vi "Configure Waveform (User Defined).vi"(0 "VISA resource name":refnum<visa-resource-name>, 1 "List Of Output Data Mode (1: New List)":i32(ring)=1 items=["Append", "New List"], 2 "Enable Trigger Output (T: Enable)":bool=TRUE, 3 "List Of Trigger Output Mode (1: New List)":i32(ring)=1 items=["Append", "New List"], 5 "Output Channel (0: Channel 1)":i32(ring) items=["Channel 1", "Channel 2"], 7 "Source Mode (1: Voltage)":i32(ring)=1 items=["Current", "Voltage"], 9 "Step Time (1E-5 seconds)":dbl=1e-05, 11 "error in (no error)":errorcluster, 12 "List Of Output Data":dbl[](array[numeric])=[0.0], 13 "Trigger Output Port (0: External1)":i32(ring) items=["External1", "External2", "External3", "External4", "External5", "External6", "External7", "External8", "External9", "External10", "External11", "External12", "External13", "External14", "Internal1", "Internal2"], 14 "List Of Trigger Output":bool[](array[boolean])=[FALSE]) -> (4 "VISA resource name out":refnum<visa-resource-name>, 15 "error out":errorcluster)   [LabVIEW 2023, in "Agilent B2900 Series.lvlib"]
doc: "Configure current or voltage user defined waveform output.\n\n<B>Note:</B>\nThis VI is only supported by Agilent models B2961A, B2962A, B2961B,B2962B,B2961C and B2962C."
uses:
  Agilent B2900 Series.lvlib
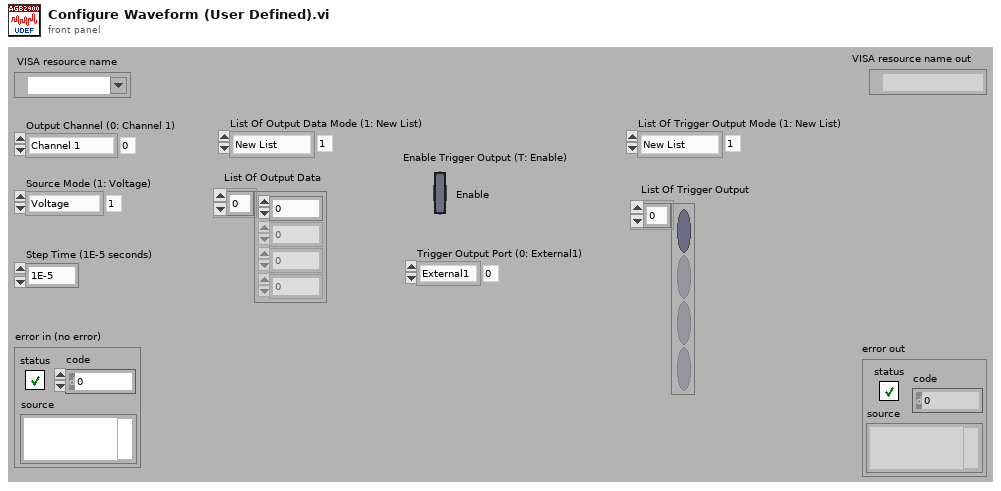
[diagram p1: front panel]
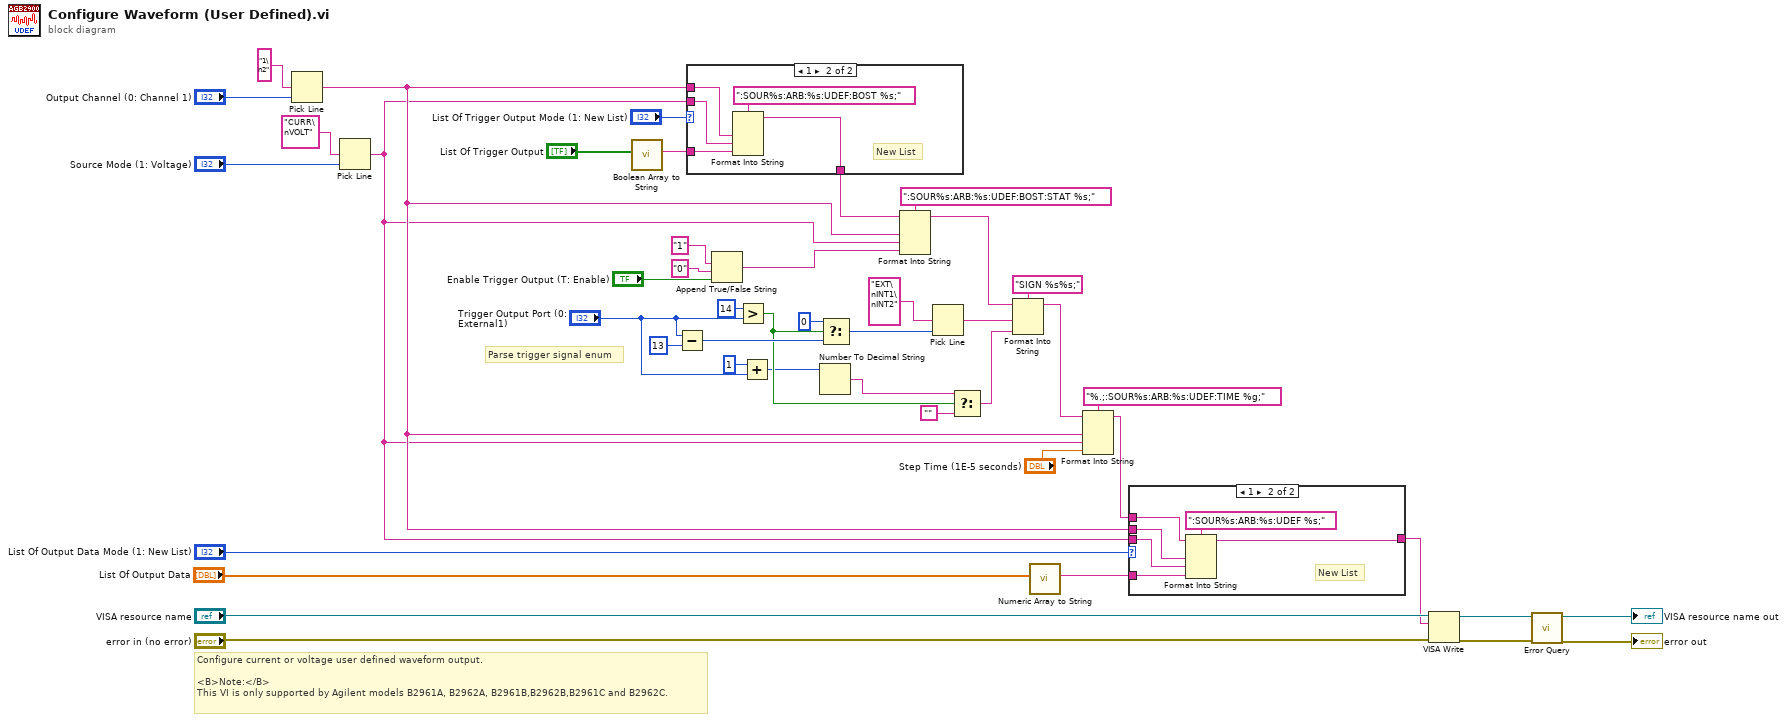
[diagram p0: block diagram]
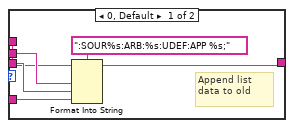
[diagram p2: hidden frame]
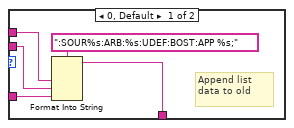
[diagram p3: hidden frame]
diagram:
  # "Parse trigger signal enum"
  # "Configure current or voltage user defined waveform output.\n\n<B>Note:</B>\nThis VI is only supported by Agilent models B2961A, B2962A, B2961B,B2962B,B2961C and B2962C."
  n1 = Pick Line(multi-line string="1\n2", line index="Output Channel (0: Channel 1)") -> (output string=w7:string)  [unwired: 1 in]
  n2 = Pick Line(multi-line string="CURR\nVOLT", line index="Source Mode (1: Voltage)") -> (output string=w6:string)  [unwired: 1 in]
  n3 = call "Boolean Array to String.vi"("List Data"="List Of Trigger Output") -> ("Result String"=w29:string)  [unwired: 10 in]
  n4 = Subtract(x="Trigger Output Port (0: External1)", y=13) -> (x-y=w23:i32)
  n5 = case shown="1" "List Of Trigger Output Mode (1: New List)" {
    tunnel: w7 -> [w49 w54]
    tunnel: w6 -> [w48 w53]
    tunnel: w29 -> [w47 w52]
    tunnel: [w46 w51] -> w9
    frame 0, Default {
      # "Append list data to old"
      n6 = Format Into String(format string=":SOUR%s:ARB:%s:UDEF:BOST:APP %s;", w49, w48, w47) -> (resulting string=w46:string)  [unwired: 2 in, 1 out]
    }
    frame 1 {
      # "New List"
      n7 = Format Into String(format string=":SOUR%s:ARB:%s:UDEF:BOST %s;", w54, w53, w52) -> (resulting string=w51:string)  [unwired: 2 in, 1 out]
    }
  }
  n8 = Append True/False String(1:"Enable Trigger Output (T: Enable)", 2:"0", 3:"1") -> (0:w10:string)  [unwired: 1 out]
  n9 = Greater?(x=14 ("y"), y="Trigger Output Port (0: External1)") -> (0:w20:bool)
  n10 = Add(x=1, y="Trigger Output Port (0: External1)") -> (x+y=w18:i32)
  n11 = Number To Decimal String(number=w18) -> (decimal integer string=w26:string)  [unwired: 1 in]
  n12 = Select(t=0, s=w20, f=w23) -> (s? t:f=w25:i32)
  n13 = Format Into String(format string=":SOUR%s:ARB:%s:UDEF:BOST:STAT %s;", initial string=w9, w7, w6, w10) -> (resulting string=w12:string)  [unwired: 1 in, 1 out]
  n14 = Pick Line(multi-line string="EXT\nINT1\nINT2", line index=w25) -> (output string=w14:string)  [unwired: 1 in]
  n15 = Select(t=w26, s=w20, f="") -> (s? t:f=w13:string)
  n16 = Format Into String(format string="SIGN %s%s;", initial string=w12, w14, w13) -> (resulting string=w11:string)  [unwired: 1 in, 1 out]
  n17 = call "Numeric Array to String.vi"("List Data"="List Of Output Data") -> ("Result String"=w16:string)  [unwired: 10 in]
  n18 = Format Into String(format string="%.;:SOUR%s:ARB:%s:UDEF:TIME %g;", initial string=w11, w7, w6, "Step Time (1E-5 seconds)") -> (resulting string=w8:string)  [unwired: 1 in, 1 out]
  n19 = case shown="1" "List Of Output Data Mode (1: New List)" {
    tunnel: w16 -> [w60 w64]
    tunnel: w7 -> [w59 w66]
    tunnel: w6 -> [w58 w65]
    tunnel: w8 -> [w57 w63]
    tunnel: [w56 w62] -> w1
    frame 0, Default {
      # "Append list data to old"
      n20 = Format Into String(format string=":SOUR%s:ARB:%s:UDEF:APP %s;", initial string=w57, w59, w58, w60) -> (resulting string=w56:string)  [unwired: 1 in, 1 out]
    }
    frame 1 {
      # "New List"
      n21 = Format Into String(format string=":SOUR%s:ARB:%s:UDEF %s;", initial string=w63, w66, w65, w64) -> (resulting string=w62:string)  [unwired: 1 in, 1 out]
    }
  }
  n22 = VISA Write(VISA resource name="VISA resource name", write buffer=w1, error in (no error)="error in (no error)") -> (VISA resource name out=w3:refnum<visa-resource-name>, error out=w2:errorcluster)  [unwired: 1 out]
  n23 = call "Error Query.vi"("error in (no error)"=w2, "VISA resource name"=w3) -> ("error out"=→"error out":errorcluster, "VISA resource name out"=→"VISA resource name out":refnum<visa-resource-name>)  [unwired: 8 out]
